vi "灯值调整停止.vi"(8 "error in (no error)":errorcluster) -> (0 "error out":errorcluster)   [LabVIEW 2016, in "斯坦道CODcr.lvlib"]
uses:
  <vilib>/Plasmionique/MB Master/MB Master.lvlib
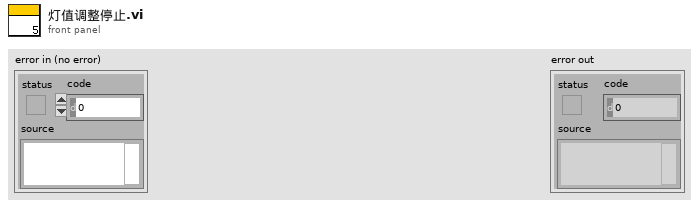
[diagram p1: front panel]
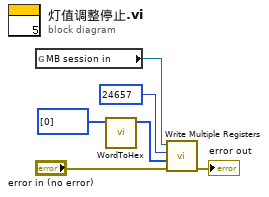
[diagram p0: block diagram]
diagram:
  n1 = global read "VAR总磷总氮全局变量.vi" "MB session in"() -> (w6:refnum<class "MB_Master.lvclass">)
  n2 = call "WordToHex.vi"("WORD"=u16[] [0]) -> ("数组"=w2:u16[])  [unwired: 10 in]
  n3 = call <vilib>:"Write Multiple Registers.vi"("error in (no error)"="error in (no error)", "values"=w2, "starting address"=u16 24657, "MB session in"=w6) -> ("error out"=→"error out":errorcluster)  [unwired: 6 in, 1 out]
